vi "max-min.vi"(10 "String 2":string, 11 "String":string) -> (0 "Sign 2":u8, 1 "Fraction":u8[](array[numeric]), 2 "Integer":u8[](array[numeric]), 3 "Sign":u8, 4 "Fraction 2":u8[](array[numeric]), 5 "Integer 2":u8[](array[numeric]))   [LabVIEW 2025]
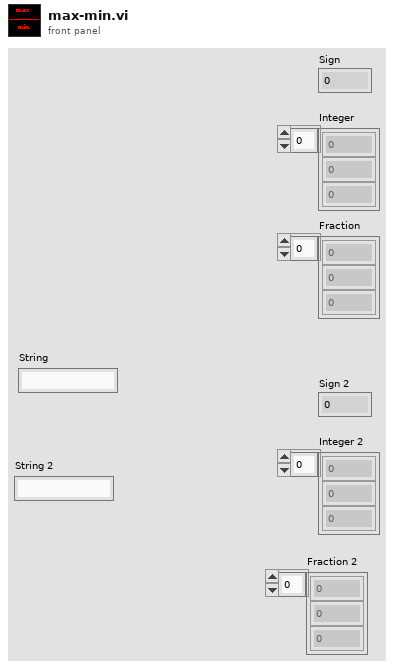
[diagram p1: front panel]
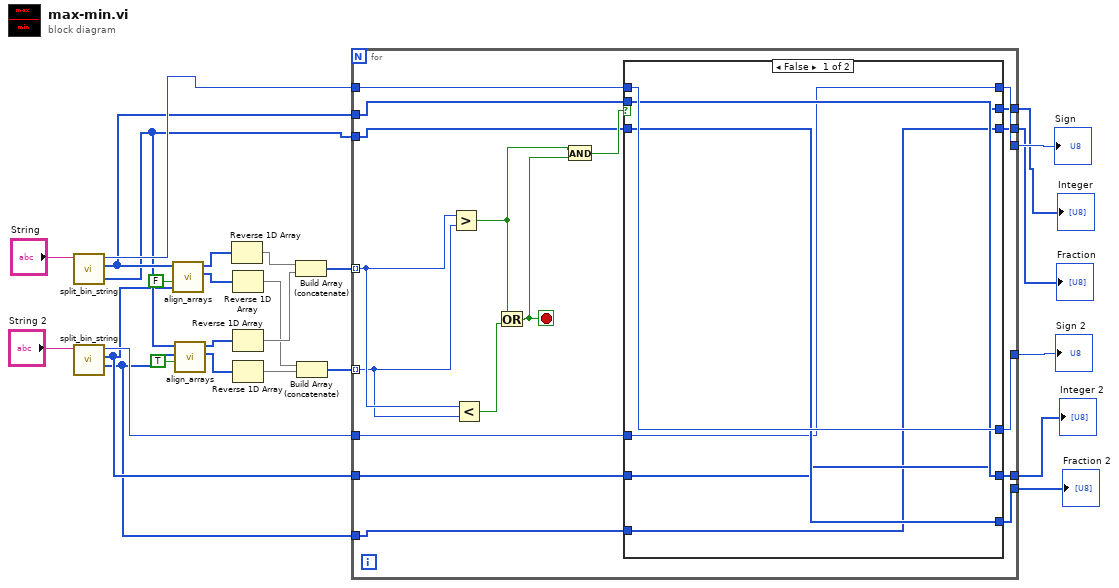
[diagram p0: block diagram]
diagram:
  n1 = call "split_bin_string.vi"("String"="String") -> ("Fraction"=w14:u8[], "Integer"=w15:u8[], "Sign"=w16:u8)  [unwired: 8 in]
  n2 = call "split_bin_string.vi"("String"="String 2") -> ("Fraction"=w11:u8[], "Integer"=w12:u8[], "Sign"=w13:u8)  [unwired: 8 in]
  n3 = call "align_arrays.vi"("IS_FRACTION"=FALSE, "Array 2"=w12, "Array"=w15) -> ("Array 4"=w23:u8[], "Array 3"=w24:u8[])  [unwired: 7 in]
  n4 = call "align_arrays.vi"("IS_FRACTION"=TRUE, "Array 2"=w11, "Array"=w14) -> ("Array 4"=w21:u8[], "Array 3"=w22:u8[])  [unwired: 7 in]
  n5 = Reverse 1D Array(array=w24) -> (reversed array=w20:u8[])
  n6 = Reverse 1D Array(array=w23) -> (reversed array=w18:u8[])
  n7 = Reverse 1D Array(array=w22) -> (reversed array=w19:u8[])
  n8 = Reverse 1D Array(array=w21) -> (reversed array=w17:u8[])
  n9 = Build Array (concatenate)(w20, w19) -> (w4:u8[])
  n10 = Build Array (concatenate)(w18, w17) -> (w3:u8[])
  n11 = for {
    tunnel: w4 -> [w44] mode=indexing
    tunnel: w3 -> [w43] mode=indexing
    tunnel: w16 -> [w38]
    tunnel: [w37] -> w10
    tunnel: w15 -> [w36]
    tunnel: [w35] -> w9
    tunnel: w14 -> [w34]
    tunnel: [w33] -> w8
    tunnel: w13 -> [w32]
    tunnel: [w31] -> w7
    tunnel: w12 -> [w30]
    tunnel: [w29] -> w6
    tunnel: w11 -> [w28]
    tunnel: [w27] -> w5
    stop <- w40 stop-if-true
    n12 = Greater?(x=w44, y=w43) -> (0:w41:bool)
    n13 = Less?(x=w44, y=w43) -> (x < y?=w42:bool)
    n14 = Or(x=w41, y=w42) -> (x .or. y?=w40:bool)
    n15 = And(x=w41, y=w40) -> (x .and. y?=w39:bool)
    n16 = case shown="False" w39 {
      tunnel: w38 -> [w50 w56]
      tunnel: [w47 w56] -> w37
      tunnel: w36 -> [w49 w55]
      tunnel: [w46 w55] -> w35
      tunnel: w34 -> [w48 w54]
      tunnel: [w45 w54] -> w33
      tunnel: w32 -> [w47 w53]
      tunnel: [w50 w53] -> w31
      tunnel: w30 -> [w46 w52]
      tunnel: [w49 w52] -> w29
      tunnel: w28 -> [w45 w51]
      tunnel: [w48 w51] -> w27
      frame False {
      }
      frame True {
      }
    }
  }
  "Sign" <- w10
  "Integer" <- w9
  "Fraction" <- w8
  "Sign 2" <- w7
  "Integer 2" <- w6
  "Fraction 2" <- w5
